vi "RAW TO STRING.vi"(10 "data out":string="5341534900480000") -> (2 "String Array":string[](array[string]), 3 "String":string)   [LabVIEW 2023]
panel:
  out "Array":string[](array[string])
  out "BArcode 2":string
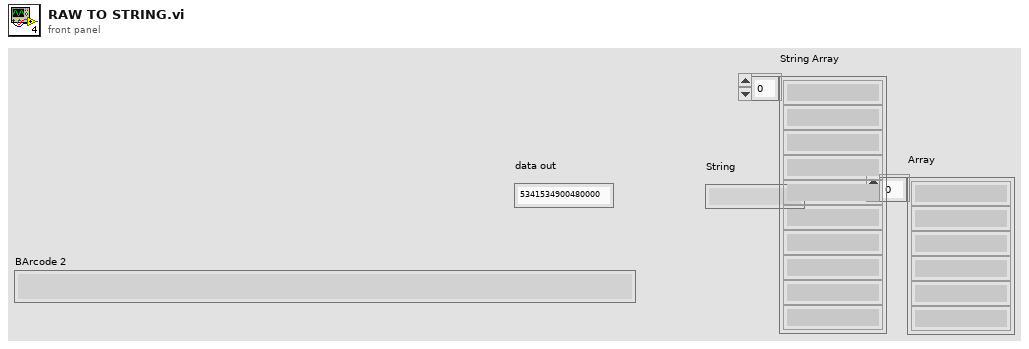
[diagram p1: front panel]
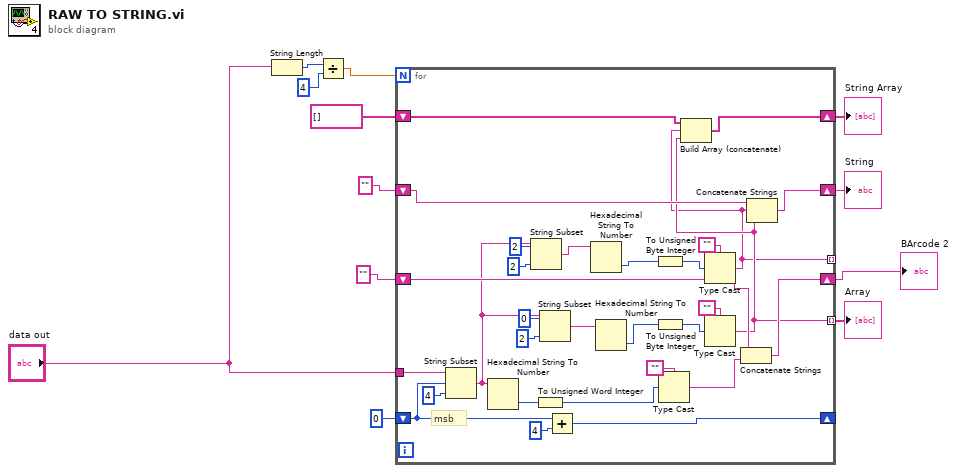
[diagram p0: block diagram]
diagram:
  n1 = String Length(string="data out") -> (length=w7:i32)
  n2 = Divide(x=w7, y=4) -> (x/y=w5:dbl)
  n3 = for {
    N: w5 -> [_]
    shift-right: [w42] -> _
    shift-left: 0 -> [w38]
    tunnel: "data out" -> [w39]
    shift-right: [w33] -> w12
    shift-left: "" -> [w34]
    tunnel: [w13] -> _ mode=indexing
    tunnel: [w14] -> w4 mode=indexing
    shift-right: [w17] -> w8
    shift-left: "" -> [w18]
    shift-right: [w15] -> w2
    shift-left: string[] [] -> [w16]
    # "msb"
    n4 = String Subset(string=w39, offset (0)=w38, length (rest)=4 ("length (rest)")) -> (substring=w27:string)
    n5 = Hexadecimal String To Number(string=w27) -> (number=w37:u32)  [unwired: 2 in, 1 out]
    n6 = String Subset(string=w27, offset (0)=2, length (rest)=2 ("length (rest)")) -> (substring=w23:string)
    n7 = To Unsigned Word Integer(number=w37) -> (unsigned 16bit integer=w36:u16)
    n8 = String Subset(string=w27, offset (0)=0, length (rest)=2 ("length (rest)")) -> (substring=w24:string)
    n9 = Add(x=w38, y=4) -> (x+y=w42:i32)
    n10 = Hexadecimal String To Number(string=w23) -> (number=w19:u32)  [unwired: 2 in, 1 out]
    n11 = Hexadecimal String To Number(string=w24) -> (number=w22:u32)  [unwired: 2 in, 1 out]
    n12 = To Unsigned Byte Integer(number=w19) -> (unsigned 8bit integer=w20:u8)
    n13 = To Unsigned Byte Integer(number=w22) -> (unsigned 8bit integer=w26:u8)
    n14 = Type Cast(type="", x=w36) -> (*(type *) &x=w32:string)
    n15 = Type Cast(type="", x=w20) -> (*(type *) &x=w13:string)
    n16 = Type Cast(type="", x=w26) -> (*(type *) &x=w14:string)
    n17 = Build Array (concatenate)(w16, w13, w14) -> (w15:string[])
    n18 = Concatenate Strings(w34, w32) -> (w33:string)
    n19 = Concatenate Strings(w18, w13, w14) -> (w17:string)
  }
  "BArcode 2" <- w12
  "String" <- w8
  "Array" <- w4
  "String Array" <- w2
